vi "ixonLiveview.vi"(11 "stop":bool) -> (1 "Left Graph":i32[][](graph) caption="On Sensor Image")   [LabVIEW 2016]
uses:
  <userlib>/atmcd64d.llb/Error Code Enum typedef.ctl
  variables/configDB.vi
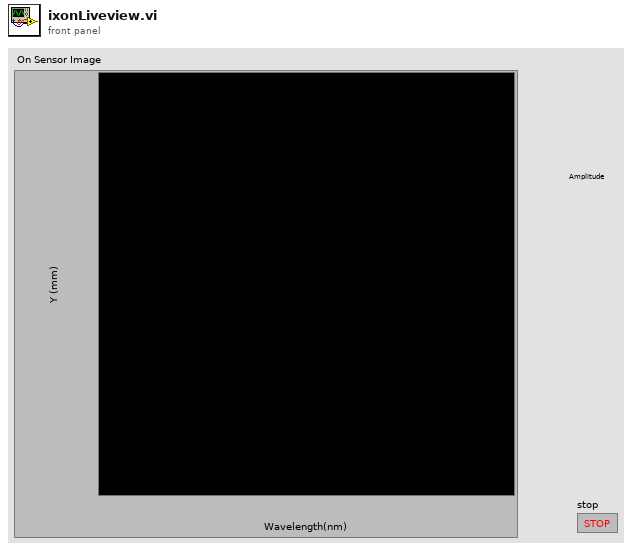
[diagram p1: front panel]
types:
  T1 = typedef "Error Code Enum typedef.ctl" = enum32{"N/A (0)", "DRV_ERROR_CODES", "DRV_SUCCESS", "DRV_VXDNOTINSTALLED", "DRV_ERROR_SCAN", "DRV_ERROR_CHECK_SUM", "DRV_ERROR_FILELOAD", "DRV_UNKNOWN_FUNC", "DRV_ERROR_VXD_INIT", "DRV_ERROR_ADDRESS", "DRV_ERROR_PAGELOCK", "DRV_ERROR_PAGEUNLOCK", "DRV_ERROR_BOARDTEST", "DRV_ERROR_ACK", "DRV_ERROR_UP_FIFO", "DRV_ERROR_PATTERN", "N/A (16)", "DRV_ACQUISITION_ERRORS", "DRV_ACQ_BUFFER", "DRV_ACQ_DOWNFIFO_FULL", "DRV_PROC_UNKONWN_INSTRUCTION", "DRV_ILLEGAL_OP_CODE", "DRV_KINETIC_TIME_NOT_MET", "DRV_ACCUM_TIME_NOT_MET", "DRV_NO_NEW_DATA", "N/A (25)", "DRV_SPOOLERROR", "N/A (27)", "N/A (28)", "N/A (29)", "N/A (30)", "N/A (31)", "N/A (32)", "DRV_TEMPERATURE_CODES", "DRV_TEMPERATURE_OFF", "DRV_TEMPERATURE_NOT_STABILIZED", "DRV_TEMPERATURE_STABILIZED", "DRV_TEMPERATURE_NOT_REACHED", "DRV_TEMPERATURE_OUT_RANGE", "DRV_TEMPERATURE_NOT_SUPPORTED", "DRV_TEMPERATURE_DRIFT", "N/A (41)", "N/A (42)", "N/A (43)", "N/A (44)", "N/A (45)", "N/A (46)", "N/A (47)", "N/A (48)", "DRV_GENERAL_ERRORS", "DRV_INVALID_AUX", "DRV_COF_NOTLOADED", "DRV_FPGAPROG", "DRV_FLEXERROR", "DRV_GPIBERROR", "N/A (55)", "N/A (56)", "N/A (57)", "N/A (58)", "N/A (59)", "N/A (60)", "N/A (61)", "N/A (62)", "N/A (63)", "DRV_DATATYPE", "DRV_DRIVER_ERRORS", "DRV_P1INVALID", "DRV_P2INVALID", "DRV_P3INVALID", "DRV_P4INVALID", "DRV_INIERROR", "DRV_COFERROR", "DRV_ACQUIRING", "DRV_IDLE", "DRV_TEMPCYCLE", "DRV_NOT_INITIALIZED", "DRV_P5INVALID", "DRV_P6INVALID", "DRV_INVALID_MODE", "DRV_INVALID_FILTER", "DRV_I2CERRORS", "DRV_I2CDEVNOTFOUND", "DRV_I2CTIMEOUT", "DRV_P7INVALID", "N/A (84)", "N/A (85)", "N/A (86)", "N/A (87)", "N/A (88)", "N/A (89)", "DRV_IOCERROR", "DRV_VRMVERSIONERROR"}
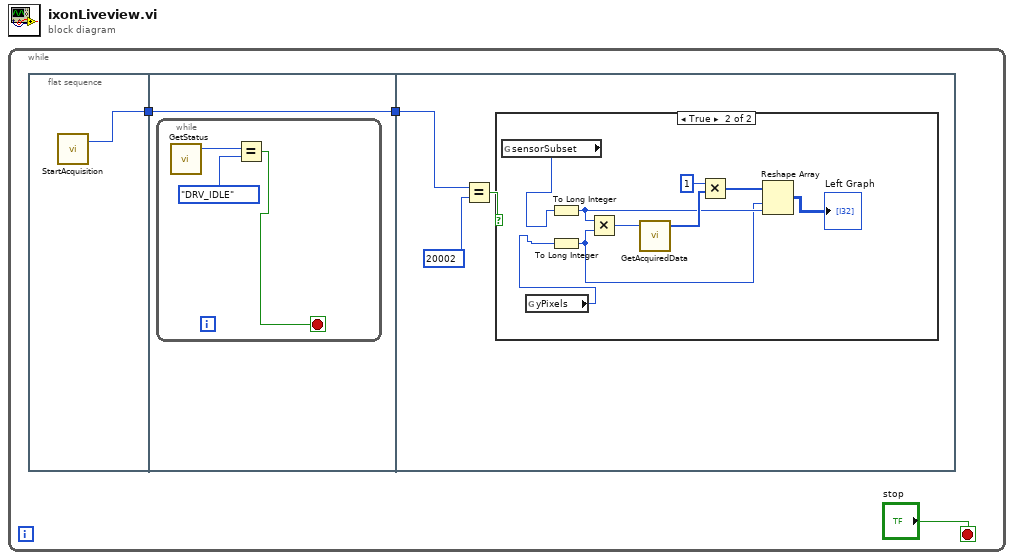
[diagram p0: block diagram]
diagram:
  n1 = while {
    stop <- "stop" stop-if-true
    n2 = flat-sequence {
      tunnel: [w4] -> w3
      tunnel: w3 -> [w5]
      tunnel: [w5] -> w2
      tunnel: w2 -> [w11]
      frame #0 {
        n3 = call <userlib>:"StartAcquisition.vi"() -> ("DLL error code"=w4:u32)  [unwired: 2 in, 1 out]
      }
      frame #1 {
        n4 = while {
          stop <- w8 stop-if-true
          n5 = call <userlib>:"GetStatus.vi"() -> ("status"=w6:T1)  [unwired: 3 in, 2 out]
          n6 = Equal?(x=w6, y=Error_Code_Enum_typedef."DRV_IDLE" ("status")) -> (x = y?=w8:bool)
        }
      }
      frame #2 {
        n7 = Equal?(x=w11, y=u32 20002) -> (x = y?=w9:bool)
        n8 = case shown="True" w9 {
          frame False {
          }
          frame True {
            n9 = global read "configDB.vi" "sensorSubset"() -> (w12:i32)
            n10 = global read "configDB.vi" "yPixels"() -> (w13:i32)
            n11 = To Long Integer(number=w12) -> (32bit integer=w16:i32)
            n12 = To Long Integer(number=w13) -> (32bit integer=w15:i32)
            n13 = Multiply(x=w16, y=w15) -> (x*y=w20:i32)
            n14 = call <userlib>:"GetAcquiredData.vi"("size"=w20) -> ("array"=w18:i32[])  [unwired: 2 in, 2 out]
            n15 = Multiply(x=1, y=w18) -> (x*y=w17:i32[])
            n16 = Reshape Array(w17, w15, w16) -> (→"Left Graph":i32[][])
          }
        }
      }
    }
  }
